vi "add tag to dictionary.vi"(8 "error in":errorcluster, 10 "system tag":refnum<class "tag descriptor.lvclass">, 11 "data dictionary in":refnum<class "data dictionary.lvclass">) -> (0 "error out":errorcluster, 3 "data dictionary out":refnum<class "data dictionary.lvclass">)   [LabVIEW 2013, in "tag bus.lvlib" / "data dictionary.lvclass"]
doc: "Adds a single tab to the data dictionary, including adding that tag to the default data table."
uses:
  data dictionary.lvclass
  tag/tag descriptor.lvclass
  tag/tag descriptor.lvclass/tag descriptor.ctl
  data dictionary.lvclass/data dictionary.ctl
  search/find insert point.vi
  table/add tag to table.vi
  tag/read default value.vi
  tag/default value polymorphs/read default value Double.vi
  tag/default value polymorphs/read default value Single.vi
  tag/default value polymorphs/read default value I64.vi
  tag/default value polymorphs/read default value I32.vi
  tag/default value polymorphs/read default value I16.vi
  tag/default value polymorphs/read default value I8.vi
  tag/default value polymorphs/read default value U64.vi
  tag/default value polymorphs/read default value U32.vi
  tag/default value polymorphs/read default value U16.vi
  tag/default value polymorphs/read default value U8.vi
  tag/default value polymorphs/read default value String.vi
  tag/default value polymorphs/read default value Boolean.vi
  tag/default value polymorphs/read default value Array of U8.vi
  tag/default value polymorphs/read default value Array of U16.vi
  tag/default value polymorphs/read default value Array of U32.vi
  tag/default value polymorphs/read default value Array of U64.vi
  tag/default value polymorphs/read default value Array of I64.vi
  tag/default value polymorphs/read default value Array of I32.vi
  tag/default value polymorphs/read default value Array of I16.vi
  tag/default value polymorphs/read default value Array of I8.vi
  tag/default value polymorphs/read default value Array of Double.vi
  tag/default value polymorphs/read default value Array of Single.vi
  tag/default value polymorphs/read default value Array of Boolean.vi
  tag/default value polymorphs/read default value Array of String.vi
  search/binary search.lvlib
  tag bus.lvlib
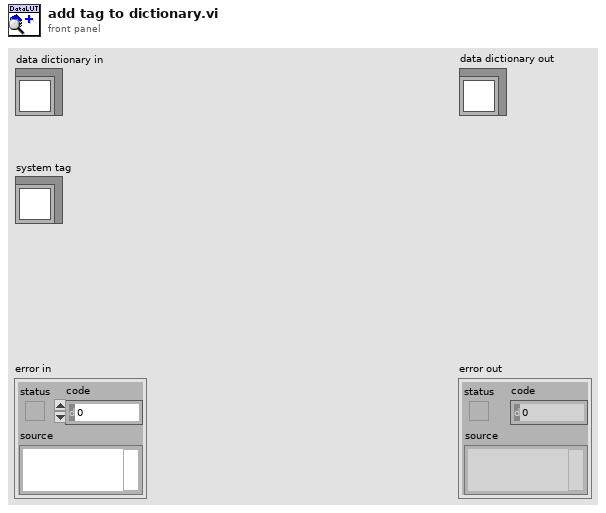
[diagram p1: front panel]
types:
  T1 = typedef "tag bus.lvlib/tag descriptor.lvclass/Data Type.ctl" = enum16{"Double", "Single", "I64", "I32", "I16", "I8", "U64", "U32", "U16", "U8", "Boolean", "String", "Array of Double", "Array of Single", "Array of I64", "Array of I32", "Array of I16", "Array of I8", "Array of U64", "Array of U32", "Array of U16", "Array of U8", "Array of Boolean", "Array of String"}
  T2 = typedef "tag bus.lvlib/binary search.lvlib/sorted list.ctl" = cluster{"sorted strings":string[], "sorted indices":i32[]}
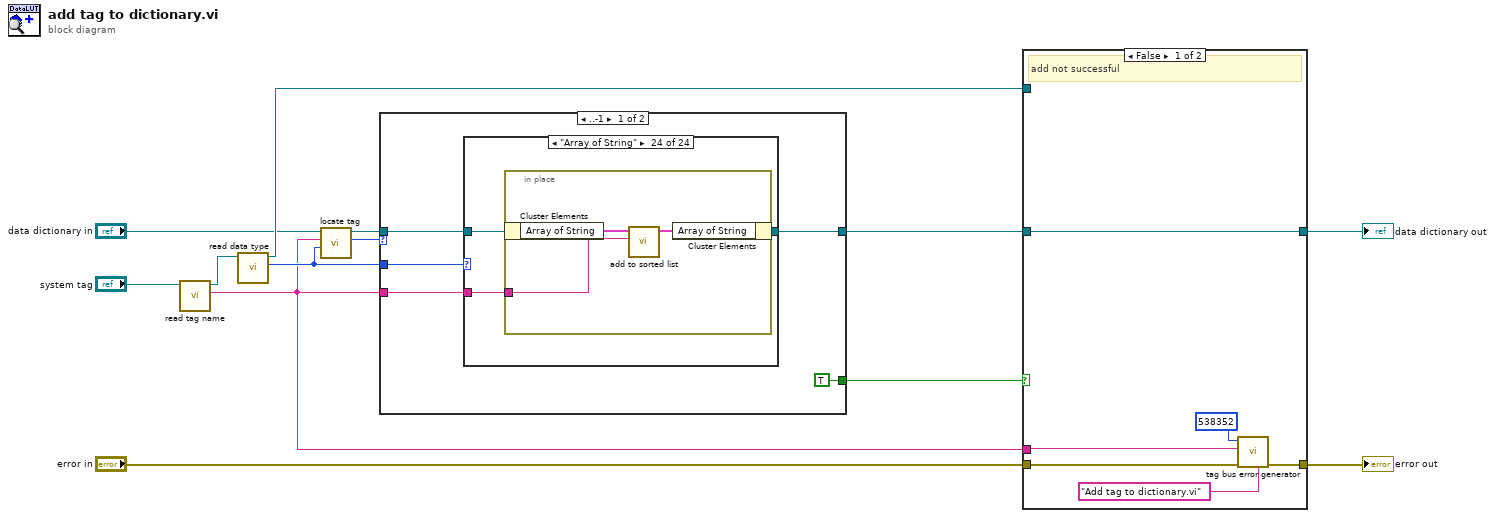
[diagram p0: block diagram]
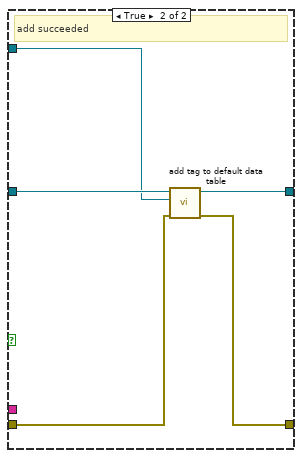
[diagram p2: hidden frame]
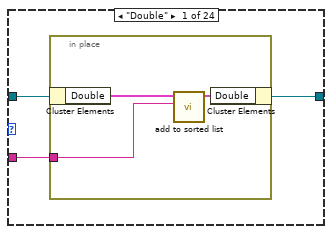
[diagram p3: hidden frame]
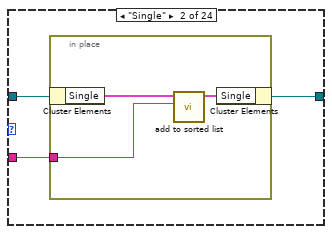
[diagram p4: hidden frame]
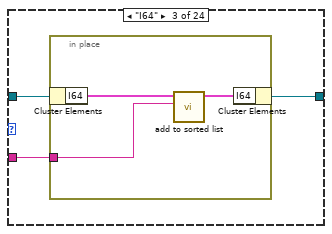
[diagram p5: hidden frame]
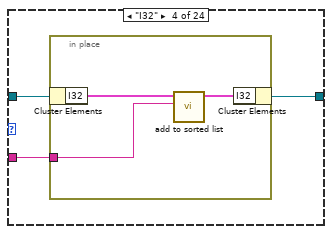
[diagram p6: hidden frame]
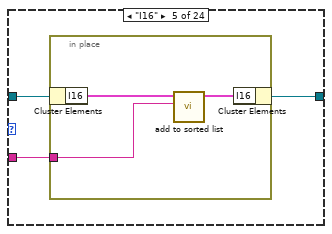
[diagram p7: hidden frame]
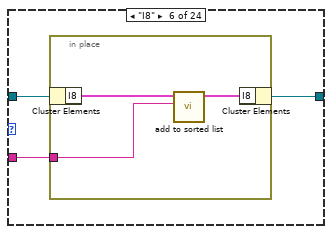
[diagram p8: hidden frame]
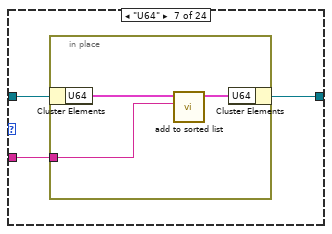
[diagram p9: hidden frame]
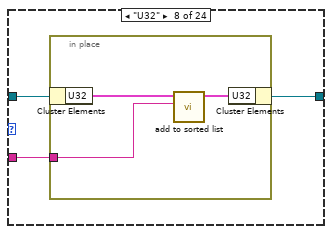
[diagram p10: hidden frame]
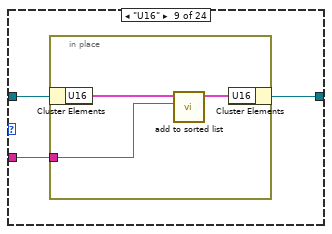
[diagram p11: hidden frame]
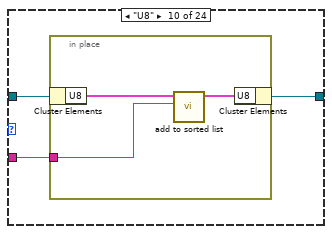
[diagram p12: hidden frame]
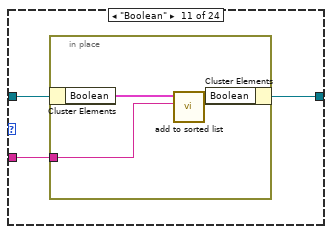
[diagram p13: hidden frame]
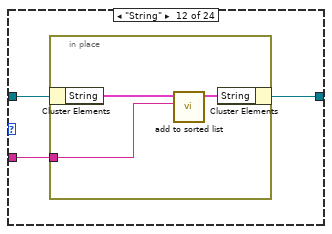
[diagram p14: hidden frame]
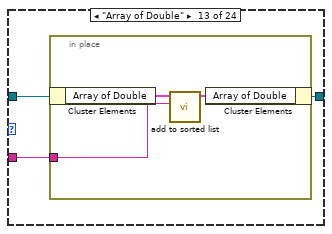
[diagram p15: hidden frame]
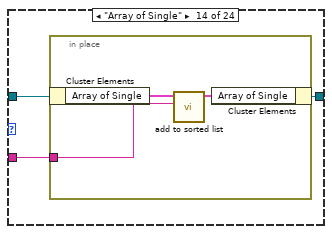
[diagram p16: hidden frame]
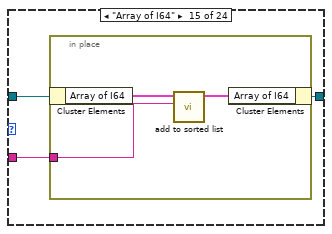
[diagram p17: hidden frame]
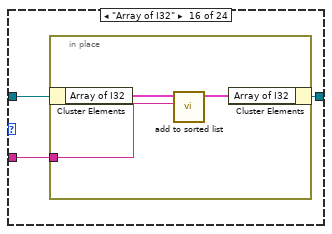
[diagram p18: hidden frame]
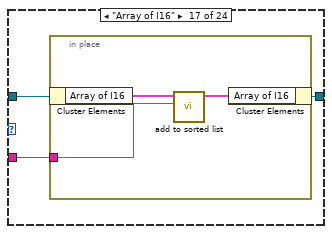
[diagram p19: hidden frame]
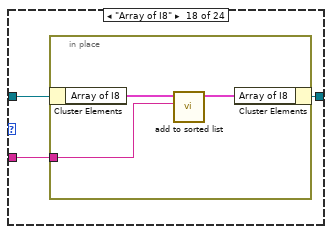
[diagram p20: hidden frame]
diagram:
  n1 = call "read tag name.vi"("system tag in"="system tag") -> ("name"=w1:string, "system tag out"=w6:refnum<class "tag descriptor.lvclass">)  [unwired: 8 in, 1 out]
  n2 = call "read data type.vi"("system tag in"=w6) -> ("data type"=w2:T1, "system tag out"=w9:refnum<class "tag descriptor.lvclass">)  [unwired: 8 in, 1 out]
  n3 = call "locate tag.vi"("data type"=w2, "name"=w1, "data dictionary in"="data dictionary in") -> ("index"=w3:i32, "data dictionary out"=w4:refnum<class "data dictionary.lvclass">)  [unwired: 6 in, 1 out]
  n4 = case shown="..-1" w3 {
    tunnel: w2 -> [w18 _]
    tunnel: w1 -> [w17 _]
    tunnel: w4 -> [w16 w164]
    tunnel: [w15 w164] -> w11
    tunnel: [TRUE FALSE] -> w7
    frame ..-1 {
      n5 = case shown="\"Array of String\"" w18 {
        tunnel: w16 -> [w21 w27 w33 w39 w45 w51 w57 w63 w69 w75 w81 w87 w93 w99 w105 w111 w117 w123 w129 w135 w141 w147 w153 w159]
        tunnel: [w20 w26 w32 w38 w44 w50 w56 w62 w68 w74 w80 w86 w92 w98 w104 w110 w116 w122 w128 w134 w140 w146 w152 w158] -> w15
        tunnel: w17 -> [w19 w25 w31 w37 w43 w49 w55 w61 w67 w73 w79 w85 w91 w97 w103 w109 w115 w121 w127 w133 w139 w145 w151 w157]
        frame "Double" {
          n6 = in-place {
            in-place-border: w19 -> [w22]
            n7 = in-place-cluster #1(w21) -> ("Double"=w24:T2)
            n8 = call "add to sorted list.vi"("string to insert"=w22, "sorted list in"=w24) -> ("sorted list out"=w23:T2)  [unwired: 9 in]
            n9 = in-place-cluster #1("Double"=w23) -> (w20:refnum<class "data dictionary.lvclass">)
          }
        }
        frame "Single" {
          n10 = in-place {
            in-place-border: w25 -> [w28]
            n11 = in-place-cluster #2(w27) -> ("Single"=w30:T2)
            n12 = call "add to sorted list.vi"("string to insert"=w28, "sorted list in"=w30) -> ("sorted list out"=w29:T2)  [unwired: 9 in]
            n13 = in-place-cluster #2("Single"=w29) -> (w26:refnum<class "data dictionary.lvclass">)
          }
        }
        frame "I64" {
          n14 = in-place {
            in-place-border: w31 -> [w34]
            n15 = in-place-cluster #3(w33) -> ("I64"=w36:T2)
            n16 = call "add to sorted list.vi"("string to insert"=w34, "sorted list in"=w36) -> ("sorted list out"=w35:T2)  [unwired: 9 in]
            n17 = in-place-cluster #3("I64"=w35) -> (w32:refnum<class "data dictionary.lvclass">)
          }
        }
        frame "I32" {
          n18 = in-place {
            in-place-border: w37 -> [w40]
            n19 = in-place-cluster #4(w39) -> ("I32"=w42:T2)
            n20 = call "add to sorted list.vi"("string to insert"=w40, "sorted list in"=w42) -> ("sorted list out"=w41:T2)  [unwired: 9 in]
            n21 = in-place-cluster #4("I32"=w41) -> (w38:refnum<class "data dictionary.lvclass">)
          }
        }
        frame "I16" {
          n22 = in-place {
            in-place-border: w43 -> [w46]
            n23 = in-place-cluster #5(w45) -> ("I16"=w48:T2)
            n24 = call "add to sorted list.vi"("string to insert"=w46, "sorted list in"=w48) -> ("sorted list out"=w47:T2)  [unwired: 9 in]
            n25 = in-place-cluster #5("I16"=w47) -> (w44:refnum<class "data dictionary.lvclass">)
          }
        }
        frame "I8" {
          n26 = in-place {
            in-place-border: w49 -> [w52]
            n27 = in-place-cluster #6(w51) -> ("I8"=w54:T2)
            n28 = call "add to sorted list.vi"("string to insert"=w52, "sorted list in"=w54) -> ("sorted list out"=w53:T2)  [unwired: 9 in]
            n29 = in-place-cluster #6("I8"=w53) -> (w50:refnum<class "data dictionary.lvclass">)
          }
        }
        frame "U64" {
          n30 = in-place {
            in-place-border: w55 -> [w58]
            n31 = in-place-cluster #7(w57) -> ("U64"=w60:T2)
            n32 = call "add to sorted list.vi"("string to insert"=w58, "sorted list in"=w60) -> ("sorted list out"=w59:T2)  [unwired: 9 in]
            n33 = in-place-cluster #7("U64"=w59) -> (w56:refnum<class "data dictionary.lvclass">)
          }
        }
        frame "U32" {
          n34 = in-place {
            in-place-border: w61 -> [w64]
            n35 = in-place-cluster #8(w63) -> ("U32"=w66:T2)
            n36 = call "add to sorted list.vi"("string to insert"=w64, "sorted list in"=w66) -> ("sorted list out"=w65:T2)  [unwired: 9 in]
            n37 = in-place-cluster #8("U32"=w65) -> (w62:refnum<class "data dictionary.lvclass">)
          }
        }
        frame "U16" {
          n38 = in-place {
            in-place-border: w67 -> [w70]
            n39 = in-place-cluster #9(w69) -> ("U16"=w72:T2)
            n40 = call "add to sorted list.vi"("string to insert"=w70, "sorted list in"=w72) -> ("sorted list out"=w71:T2)  [unwired: 9 in]
            n41 = in-place-cluster #9("U16"=w71) -> (w68:refnum<class "data dictionary.lvclass">)
          }
        }
        frame "U8" {
          n42 = in-place {
            in-place-border: w73 -> [w76]
            n43 = in-place-cluster #10(w75) -> ("U8"=w78:T2)
            n44 = call "add to sorted list.vi"("string to insert"=w76, "sorted list in"=w78) -> ("sorted list out"=w77:T2)  [unwired: 9 in]
            n45 = in-place-cluster #10("U8"=w77) -> (w74:refnum<class "data dictionary.lvclass">)
          }
        }
        frame "Boolean" {
          n46 = in-place {
            in-place-border: w79 -> [w82]
            n47 = in-place-cluster #11(w81) -> ("Boolean"=w84:T2)
            n48 = call "add to sorted list.vi"("string to insert"=w82, "sorted list in"=w84) -> ("sorted list out"=w83:T2)  [unwired: 9 in]
            n49 = in-place-cluster #11("Boolean"=w83) -> (w80:refnum<class "data dictionary.lvclass">)
          }
        }
        frame "String" {
          n50 = in-place {
            in-place-border: w85 -> [w88]
            n51 = in-place-cluster #12(w87) -> ("String"=w90:T2)
            n52 = call "add to sorted list.vi"("string to insert"=w88, "sorted list in"=w90) -> ("sorted list out"=w89:T2)  [unwired: 9 in]
            n53 = in-place-cluster #12("String"=w89) -> (w86:refnum<class "data dictionary.lvclass">)
          }
        }
        frame "Array of Double" {
          n54 = in-place {
            in-place-border: w91 -> [w94]
            n55 = in-place-cluster #13(w93) -> ("Array of Double"=w96:T2)
            n56 = call "add to sorted list.vi"("string to insert"=w94, "sorted list in"=w96) -> ("sorted list out"=w95:T2)  [unwired: 9 in]
            n57 = in-place-cluster #13("Array of Double"=w95) -> (w92:refnum<class "data dictionary.lvclass">)
          }
        }
        frame "Array of Single" {
          n58 = in-place {
            in-place-border: w97 -> [w100]
            n59 = in-place-cluster #14(w99) -> ("Array of Single"=w102:T2)
            n60 = call "add to sorted list.vi"("string to insert"=w100, "sorted list in"=w102) -> ("sorted list out"=w101:T2)  [unwired: 9 in]
            n61 = in-place-cluster #14("Array of Single"=w101) -> (w98:refnum<class "data dictionary.lvclass">)
          }
        }
        frame "Array of I64" {
          n62 = in-place {
            in-place-border: w103 -> [w106]
            n63 = in-place-cluster #15(w105) -> ("Array of I64"=w108:T2)
            n64 = call "add to sorted list.vi"("string to insert"=w106, "sorted list in"=w108) -> ("sorted list out"=w107:T2)  [unwired: 9 in]
            n65 = in-place-cluster #15("Array of I64"=w107) -> (w104:refnum<class "data dictionary.lvclass">)
          }
        }
        frame "Array of I32" {
          n66 = in-place {
            in-place-border: w109 -> [w112]
            n67 = in-place-cluster #16(w111) -> ("Array of I32"=w114:T2)
            n68 = call "add to sorted list.vi"("string to insert"=w112, "sorted list in"=w114) -> ("sorted list out"=w113:T2)  [unwired: 9 in]
            n69 = in-place-cluster #16("Array of I32"=w113) -> (w110:refnum<class "data dictionary.lvclass">)
          }
        }
        frame "Array of I16" {
          n70 = in-place {
            in-place-border: w115 -> [w118]
            n71 = in-place-cluster #17(w117) -> ("Array of I16"=w120:T2)
            n72 = call "add to sorted list.vi"("string to insert"=w118, "sorted list in"=w120) -> ("sorted list out"=w119:T2)  [unwired: 9 in]
            n73 = in-place-cluster #17("Array of I16"=w119) -> (w116:refnum<class "data dictionary.lvclass">)
          }
        }
        frame "Array of I8" {
          n74 = in-place {
            in-place-border: w121 -> [w124]
            n75 = in-place-cluster #18(w123) -> ("Array of I8"=w126:T2)
            n76 = call "add to sorted list.vi"("string to insert"=w124, "sorted list in"=w126) -> ("sorted list out"=w125:T2)  [unwired: 9 in]
            n77 = in-place-cluster #18("Array of I8"=w125) -> (w122:refnum<class "data dictionary.lvclass">)
          }
        }
        frame "Array of U64" {
          n78 = in-place {
            in-place-border: w127 -> [w130]
            n79 = in-place-cluster #19(w129) -> ("Array of U64"=w132:T2)
            n80 = call "add to sorted list.vi"("string to insert"=w130, "sorted list in"=w132) -> ("sorted list out"=w131:T2)  [unwired: 9 in]
            n81 = in-place-cluster #19("Array of U64"=w131) -> (w128:refnum<class "data dictionary.lvclass">)
          }
        }
        frame "Array of U32" {
          n82 = in-place {
            in-place-border: w133 -> [w136]
            n83 = in-place-cluster #20(w135) -> ("Array of U32"=w138:T2)
            n84 = call "add to sorted list.vi"("string to insert"=w136, "sorted list in"=w138) -> ("sorted list out"=w137:T2)  [unwired: 9 in]
            n85 = in-place-cluster #20("Array of U32"=w137) -> (w134:refnum<class "data dictionary.lvclass">)
          }
        }
        frame "Array of U16" {
          n86 = in-place {
            in-place-border: w139 -> [w142]
            n87 = in-place-cluster #21(w141) -> ("Array of U16"=w144:T2)
            n88 = call "add to sorted list.vi"("string to insert"=w142, "sorted list in"=w144) -> ("sorted list out"=w143:T2)  [unwired: 9 in]
            n89 = in-place-cluster #21("Array of U16"=w143) -> (w140:refnum<class "data dictionary.lvclass">)
          }
        }
        frame "Array of U8" {
          n90 = in-place {
            in-place-border: w145 -> [w148]
            n91 = in-place-cluster #22(w147) -> ("Array of U8"=w150:T2)
            n92 = call "add to sorted list.vi"("string to insert"=w148, "sorted list in"=w150) -> ("sorted list out"=w149:T2)  [unwired: 9 in]
            n93 = in-place-cluster #22("Array of U8"=w149) -> (w146:refnum<class "data dictionary.lvclass">)
          }
        }
        frame "Array of Boolean" {
          n94 = in-place {
            in-place-border: w151 -> [w154]
            n95 = in-place-cluster #23(w153) -> ("Array of Boolean"=w156:T2)
            n96 = call "add to sorted list.vi"("string to insert"=w154, "sorted list in"=w156) -> ("sorted list out"=w155:T2)  [unwired: 9 in]
            n97 = in-place-cluster #23("Array of Boolean"=w155) -> (w152:refnum<class "data dictionary.lvclass">)
          }
        }
        frame "Array of String" {
          n98 = in-place {
            in-place-border: w157 -> [w160]
            n99 = in-place-cluster #24(w159) -> ("Array of String"=w162:T2)
            n100 = call "add to sorted list.vi"("string to insert"=w160, "sorted list in"=w162) -> ("sorted list out"=w161:T2)  [unwired: 9 in]
            n101 = in-place-cluster #24("Array of String"=w161) -> (w158:refnum<class "data dictionary.lvclass">)
          }
        }
      }
    }
    frame 0.. {
    }
  }
  n102 = case shown="False" w7 {
    tunnel: "error in" -> [w170 w174]
    tunnel: [w169 w173] -> w13
    tunnel: w1 -> [w167 _]
    tunnel: w11 -> [w166 w175]
    tunnel: [w166 w172] -> w10
    tunnel: w9 -> [_ w171]
    frame False {
      # "add not successful"
      n103 = call "tag bus error generator.vi"("error in"=w170, "source"="Add tag to dictionary.vi", "append error message"=w167, "error code (0)"=538352) -> ("error out"=w169:errorcluster)  [unwired: 5 in]
    }
    frame True {
      # "add succeeded"
      n104 = call "add tag to default data table.vi"("error in"=w174, "system tag"=w171, "data dictionary in"=w175) -> ("error out"=w173:errorcluster, "data dictionary out"=w172:refnum<class "data dictionary.lvclass">)  [unwired: 7 in]
    }
  }
  "error out" <- w13
  "data dictionary out" <- w10
